vi "SMCcontrol.vi"() -> ()   [LabVIEW 2011]
panel:
  out "Axis 2 (y axis)":dbl format="%.6f"
  in  "Axis in":i32=1
  in  "forward":bool
  in  "Relative Step Size":dbl
  in  "back":bool
  in  "move abs":bool
  in  "Absolute Target":dbl
  out "Axis 1 x axis":dbl format="%.6f"
  in  "stop":bool
  in  "VISA Handle in":refnum<visa-resource-name>
  # "+x moves sample to the left\n+y moves sample up\nMax range for y is 9\nMax range for x is 24"
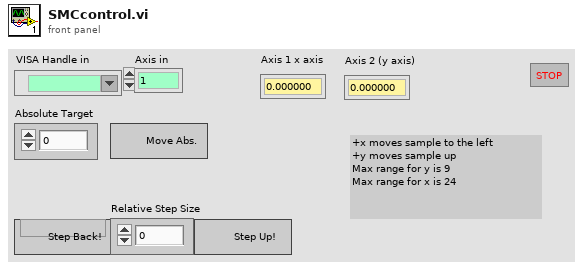
[diagram p1: front panel]
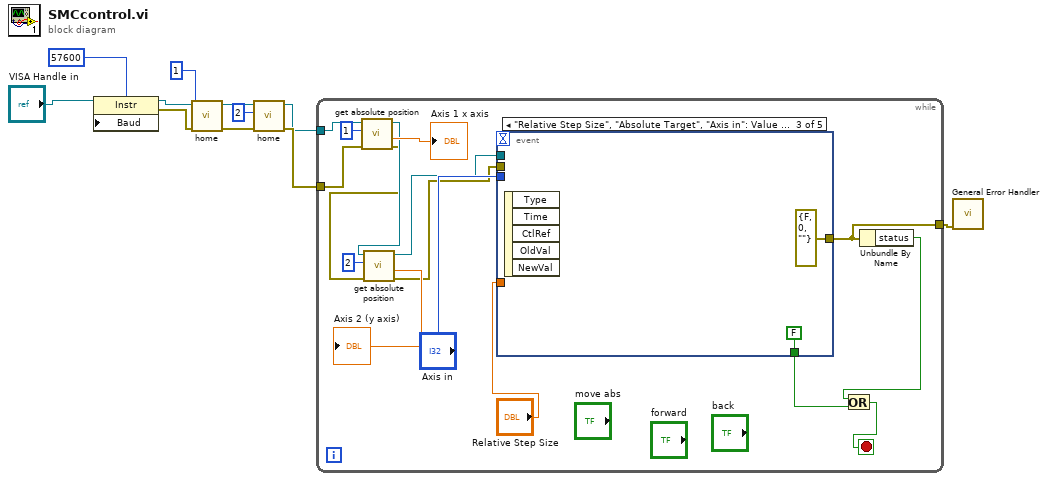
[diagram p0: block diagram]
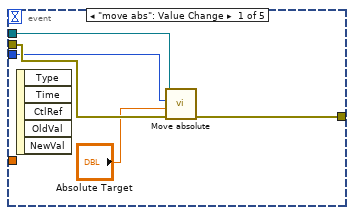
[diagram p2: hidden frame]
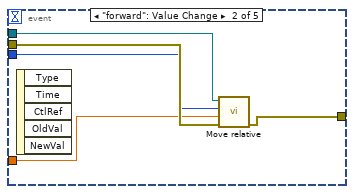
[diagram p3: hidden frame]
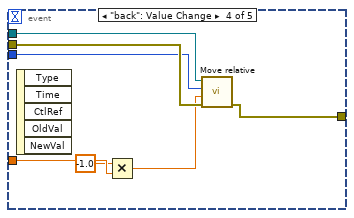
[diagram p4: hidden frame]
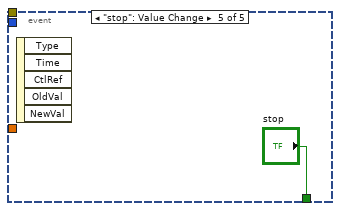
[diagram p5: hidden frame]
diagram:
  n1 = property class="Instr"(reference="VISA Handle in", "Baud"=u32 57600 ("Serial Settings:Baud Rate")) -> (reference out=w3:refnum<visa-resource-name>, error out=w2:errorcluster)  [unwired: 1 in]
  n2 = call "home.vi"("error in"=w2, "Axis in"=1, "VISA Handle in"=w3) -> ("error out"=w11:errorcluster, "VISA Handle out"=w8:refnum<visa-resource-name>)  [unwired: 3 in, 2 out]
  n3 = call "home.vi"("error in"=w11, "Axis in"=2, "VISA Handle in"=w8) -> ("error out"=w10:errorcluster, "VISA Handle out"=w9:refnum<visa-resource-name>)  [unwired: 3 in, 2 out]
  n4 = while {
    tunnel: w9 -> [w27]
    tunnel: w10 -> [w25]
    tunnel: [w13] -> w5
    stop <- w14 stop-if-true
    n5 = call "get absolute position.vi"("error in"=w25, "Axis in"=1, "VISA Handle in"=w27) -> ("error out"=w18:errorcluster, "Target position (units)"=→"Axis 1 x axis":dbl, "VISA Handle out"=w19:refnum<visa-resource-name>)  [unwired: 2 in, 2 out]
    n6 = call "get absolute position.vi"("error in"=w18, "Axis in"=2, "VISA Handle in"=w19) -> ("error out"=w17:errorcluster, "Target position (units)"=→"Axis 2 (y axis)":dbl, "VISA Handle out"=w12:refnum<visa-resource-name>)  [unwired: 2 in, 2 out]
    n7 = event shown="[2] \"Relative Step Size\", \"Absolute Target\", \"Axis in\": Value Change" {
      selector: _ -> [_ _ _ _ _]
      dyn-events: _ -> [_ _ _ _ _]
      timeout: _ -> [_ _ _ _ _]
      tunnel: w17 -> [w32 w37 _ w46 _]
      tunnel: [w30 w35 errorcluster {"status"=FALSE, "code"=0, "source"=""} ("error out") w42 _] -> w13
      tunnel: "Relative Step Size" -> [_ w36 _ w45 _]
      tunnel: [_ _ FALSE ("stop") _ "stop"] -> w15
      tunnel: "Axis in" -> [w29 w34 _ w41 _]
      tunnel: w12 -> [w28 w33 _ w40 _]
      event "move abs": Value Change {
        n8 = event-data() -> ()  [unwired: 1 in, 5 out]
        n9 = call "Move absolute.vi"("error in"=w32, "New target position (units)"="Absolute Target", "Axis in"=w29, "VISA Handle in"=w28) -> ("error out"=w30:errorcluster)  [unwired: 2 in, 3 out]
      }
      event "forward": Value Change {
        n10 = event-data() -> ()  [unwired: 1 in, 5 out]
        n11 = call "Move relative.vi"("error in"=w37, "Displacement (units)"=w36, "Axis in"=w34, "VISA Handle in"=w33) -> ("error out"=w35:errorcluster)  [unwired: 2 in, 3 out]
      }
      event "Relative Step Size", "Absolute Target", "Axis in": Value Change {
        n12 = event-data() -> ()  [unwired: 1 in, 5 out]
      }
      event "back": Value Change {
        n13 = event-data() -> ()  [unwired: 1 in, 5 out]
        n14 = Multiply(x=-1.0, y=w45) -> (x*y=w43:dbl)
        n15 = call "Move relative.vi"("error in"=w46, "Displacement (units)"=w43, "Axis in"=w41, "VISA Handle in"=w40) -> ("error out"=w42:errorcluster)  [unwired: 2 in, 3 out]
      }
      event "stop": Value Change {
        n16 = event-data() -> ()  [unwired: 1 in, 5 out]
      }
    }
    n17 = Unbundle By Name(w13) -> ("status"=w16:bool)
    n18 = Or(x=w16, y=w15) -> (x .or. y?=w14:bool)
  }
  n19 = call <vilib>:"General Error Handler.vi"("error in (no error)"=w5) -> ()  [unwired: 10 in, 5 out]
